vi "Channel Measurement Marker Query Bandwidth.vi"(8 "error in (no error)":errorcluster {"code" format="%.0x"}, 9 "RepCapIdentifier":string, 11 "instrument handle":refnum<k15>) -> (0 "error out":errorcluster {"code" format="%.0x"}, 1 "pCenterFreqVal":dbl, 2 "pBandWidthVal":dbl, 3 "instrument handle out":refnum<k15>, 4 "pQVal":dbl, 5 "pLossVal":dbl)   [LabVIEW 2014, in "Agilent NA.lvlib"]
doc: "Method QueryBandwidth"
uses:
  Agilent NA.lvlib
  AgNA.dll
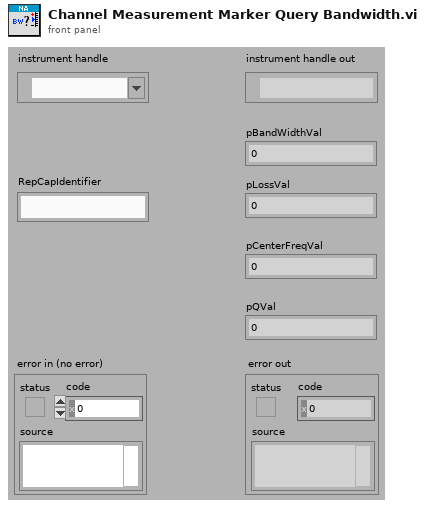
[diagram p1: front panel]
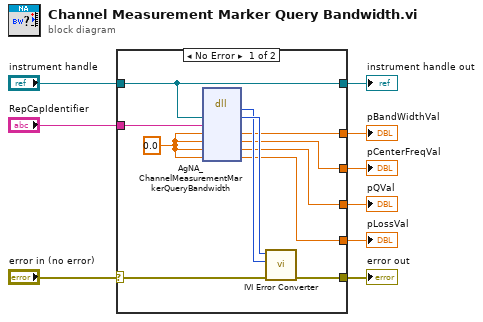
[diagram p0: block diagram]
diagram:
  n1 = case shown="No Error" "error in (no error)" {
    selector: "error in (no error)" -> [w18 w22]
    tunnel: [w17 w22] -> w9
    tunnel: "RepCapIdentifier" -> [w16 _]
    tunnel: [w15 _] -> w6
    tunnel: [w14 _] -> w5
    tunnel: [w13 _] -> w4
    tunnel: [w12 _] -> w3
    tunnel: [w11 w21] -> w2
    tunnel: "instrument handle" -> [w11 w21]
    frame No Error {
      w10 = 0.0 ("pBandWidthVal")
      n2 = dll-call lib="AgNA**.dll" fn="AgNA_ChannelMeasurementMarkerQueryBandwidth"("Vi"=w11, "RepCapIdentifier"=w16, "pBandWidthVal"=w10, "pCenterFreqVal"=w10, "pQVal"=w10, "pLossVal"=w10) -> (w19:i32, "Vi"=w20:u32, "pBandWidthVal"=w15:dbl, "pCenterFreqVal"=w14:dbl, "pQVal"=w13:dbl, "pLossVal"=w12:dbl)  [unwired: 4 in, 2 out]
      n3 = call "IVI Error Converter.vi"("error in (no error)"=w18, "IVI error code (0)"=w19, "instrument handle"=w20) -> ("error out"=w17:errorcluster)  [unwired: 7 in, 1 out]
    }
    frame Error {
    }
  }
  "error out" <- w9
  "instrument handle out" <- w2
  "pBandWidthVal" <- w6
  "pCenterFreqVal" <- w5
  "pQVal" <- w4
  "pLossVal" <- w3
